vi "Stepper System Control.vi"() -> ()   [LabVIEW 2018]
uses:
  <vilib>/LabVIEW Interface for Arduino/LabVIEW Interface for Arduino.lvlib
panel:
  in  "zero bottom":bool
  in  "stop program":bool
  in  "return to start":bool
  out "Current position":dbl
  in  "move":bool
  in  "Distance to go (mm)":dbl
  in  "Set speed (steps/s)":dbl min=0.0 max=140.0
  in  "turn":bool
  in  "Serial Port":refnum<visa-resource-name>
  in  "zero top":bool
  # "Returns to lowest position."
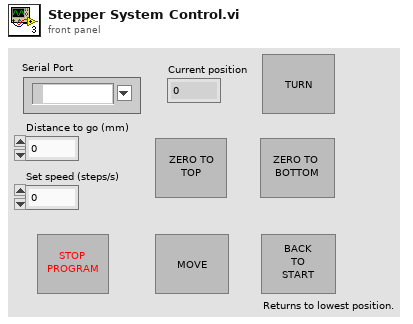
[diagram p1: front panel]
types:
  T1 = typedef "LabVIEW Interface for Arduino.lvlib/Arduino Resource.ctl" = cluster{"VISA resource":refnum<visa-resource-name>, "Board Type":T2, "Connection Type":enum8{"USB / Serial"}, "Bytes Per Packet (15)":u8}
  T2 = typedef "LabVIEW Interface for Arduino.lvlib/Board Type.ctl" = enum16{"Uno", "Dimuelanove w/Atmega 328", "Mega 2560"}
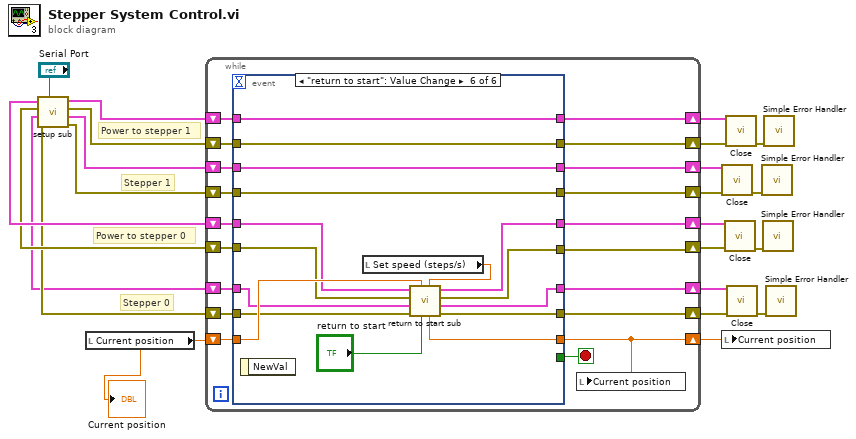
[diagram p0: block diagram]
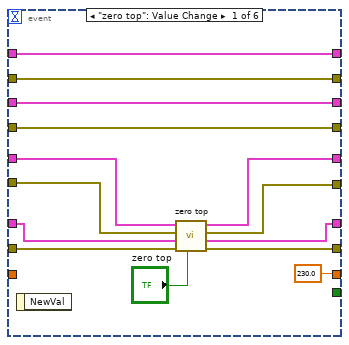
[diagram p2: hidden frame]
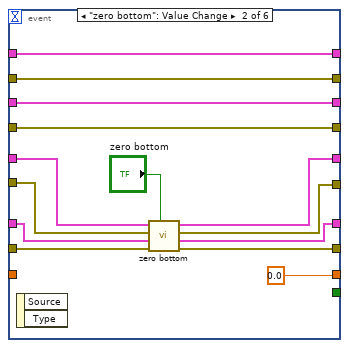
[diagram p3: hidden frame]
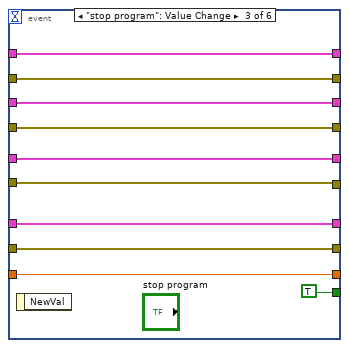
[diagram p4: hidden frame]
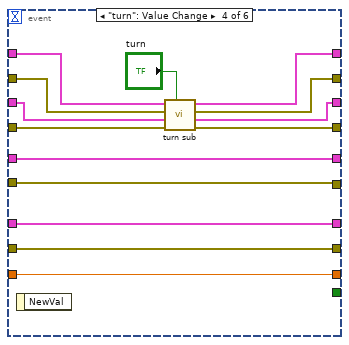
[diagram p5: hidden frame]
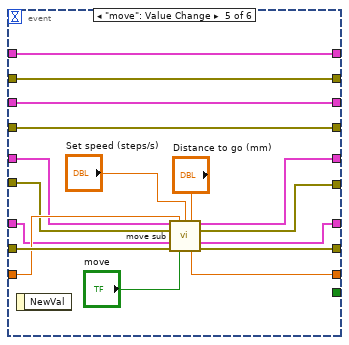
[diagram p6: hidden frame]
diagram:
  # "Power to stepper 0"
  # "Power to stepper 1"
  # "Stepper 1"
  # "Stepper 0"
  n1 = call "setup sub.vi"("Serial port in"="Serial Port") -> ("Stepper 1 error out"=w9:errorcluster, "Stepper 1 out"=w8:T1, "Pin 8 error out"=w1:errorcluster, "Pin 8 out"=w2:T1, "Stepper 0 error out"=w4:errorcluster, "Stepper 0 out"=w3:T1, "Pin 2 error out"=w6:errorcluster, "Pin 2 out"=w7:T1)  [unwired: 3 in]
  n2 = local read "Current position"() -> (w13:dbl)
  "Current position" <- w13
  n3 = while {
    shift-right: [w32] -> w16
    shift-left: w3 -> [w42]
    shift-right: [w33] -> w17
    shift-left: w4 -> [w41]
    shift-right: [w31] -> w15
    shift-left: w8 -> [w40]
    shift-right: [w34] -> w18
    shift-left: w9 -> [w39]
    shift-right: [w36] -> w20
    shift-left: w7 -> [w38]
    shift-right: [w35] -> w19
    shift-left: w6 -> [w37]
    shift-right: [w28] -> w14
    shift-left: w13 -> [w30]
    shift-right: [w27] -> w11
    shift-left: w2 -> [w24]
    shift-right: [w26] -> w10
    shift-left: w1 -> [w25]
    stop <- w29 stop-if-true
    n4 = event shown="[5] \"return to start\": Value Change" {
      selector: _ -> [_ _ _ _ _ _]
      dyn-events: _ -> [_ _ _ _ _ _]
      timeout: _ -> [_ _ _ _ _ _]
      tunnel: w42 -> [w53 w68 w74 w88 w101 w124]
      tunnel: w41 -> [w55 w69 w73 w87 w110 w123]
      tunnel: w40 -> [w51 w59 w77 w91 w108 w120]
      tunnel: w39 -> [w50 w60 w76 w94 w107 w119]
      tunnel: w38 -> [w48 w65 w79 w86 w104 w115]
      tunnel: w37 -> [w49 w66 w78 w85 w105 w116]
      tunnel: [w46 w64 w79 w86 w106 w117] -> w36
      tunnel: [w47 w63 w78 w85 w98 w118] -> w35
      tunnel: [w50 w60 w76 w92 w107 w119] -> w34
      tunnel: [w54 w70 w73 w87 w99 w121] -> w33
      tunnel: [w52 w67 w74 w88 w100 w122] -> w32
      tunnel: [w51 w59 w77 w90 w108 w120] -> w31
      tunnel: w30 -> [_ _ w75 w89 w109 w125]
      tunnel: [230.0 0.0 w75 w89 w97 w126] -> w28
      tunnel: [_ _ TRUE _ _ _] -> w29
      tunnel: [w44 w57 w71 w84 w95 w112] -> w27
      tunnel: [w45 w58 w72 w83 w96 w113] -> w26
      tunnel: w25 -> [w45 w58 w72 w82 w96 w113]
      tunnel: w24 -> [w44 w57 w71 w81 w95 w112]
      event "zero top": Value Change {
        n5 = event-data() -> ()  [unwired: 1 in, 1 out]
        n6 = call "zero top.vi"("zero"="zero top", "Stepper 0 error in"=w55, "Stepper 0 in"=w53, "Pin 2 error in"=w49, "Pin 2 in"=w48) -> ("Stepper 0 error out"=w54:errorcluster, "Stepper 0 out"=w52:T1, "Pin 2 error out"=w47:errorcluster, "Pin 2 out"=w46:T1)  [unwired: 3 in]
      }
      event "zero bottom": Value Change {
        n7 = event-data() -> ()  [unwired: 1 in, 2 out]
        n8 = call "zero bottom.vi"("zero"="zero bottom", "Stepper 0 error in"=w69, "Stepper 0 in"=w68, "Pin 2 error in"=w66, "Pin 2 in"=w65) -> ("Stepper 0 error out"=w70:errorcluster, "Stepper 0 out"=w67:T1, "Pin 2 error out"=w63:errorcluster, "Pin 2 out"=w64:T1)  [unwired: 3 in]
      }
      event "stop program": Value Change {
        n9 = event-data() -> ()  [unwired: 1 in, 1 out]
      }
      event "turn": Value Change {
        n10 = event-data() -> ()  [unwired: 1 in, 1 out]
        n11 = call "turn sub.vi"("turn Button"="turn", "Stepper 1 error in"=w94, "Stepper 1 in"=w91, "Pin 12 error in"=w82, "Pin 12 in"=w81) -> ("Stepper 1 error out"=w92:errorcluster, "Stepper 1 out"=w90:T1, "Pin 12 error out"=w83:errorcluster, "Pin 12 out"=w84:T1)  [unwired: 3 in]
      }
      event "move": Value Change {
        n12 = event-data() -> ()  [unwired: 1 in, 1 out]
        n13 = call "move sub.vi"("Pin 2 in"=w104, "Current position in"=w109, "Set speed"="Set speed (steps/s)", "mm to go"="Distance to go (mm)", "Pin 2 error in"=w105, "Stepper 0 in"=w101, "Stepper 0 error in"=w110, "Move"="move") -> ("Pin 2 out"=w106:T1, "Pin 2 error out"=w98:errorcluster, "Stepper 0 out"=w100:T1, "Current position out"=w97:dbl, "Stepper 0 error out"=w99:errorcluster)  [unwired: 3 in]
      }
      event "return to start": Value Change {
        n14 = event-data() -> ()  [unwired: 1 in, 1 out]
        n15 = local read "Set speed (steps/s)"() -> (w114:dbl)
        n16 = call "return to start sub.vi"("Set speed"=w114, "Return to start"="return to start", "Current position in"=w125, "Stepper 0 error in"=w123, "Stepper 0 in"=w124, "Pin 2 error in"=w116, "Pin 2 in"=w115) -> ("Stepper 0 error out"=w121:errorcluster, "Stepper 0 out"=w122:T1, "Pin 2 error out"=w118:errorcluster, "Pin 2 out"=w117:T1, "Current position out"=w126:dbl)
      }
    }
    n17 = local write "Current position"(w28) -> ()
  }
  n18 = call <vilib>:"Close.vi"("Arduino Resource"=w15, "error in"=w18) -> ("error out"=w22:errorcluster)  [unwired: 13 in]
  n19 = local write "Current position"(w14) -> ()
  n20 = call <vilib>:"Close.vi"("Arduino Resource"=w20, "error in"=w19) -> ("error out"=w21:errorcluster)  [unwired: 13 in]
  n21 = call <vilib>:"Close.vi"("Arduino Resource"=w11, "error in"=w10) -> ("error out"=w12:errorcluster)  [unwired: 13 in]
  n22 = call <vilib>:"Close.vi"("Arduino Resource"=w16, "error in"=w17) -> ("error out"=w23:errorcluster)  [unwired: 13 in]
  n23 = call <vilib>:"Simple Error Handler.vi"("error in (no error)"=w22) -> ()  [unwired: 4 in, 5 out]
  n24 = call <vilib>:"Simple Error Handler.vi"("error in (no error)"=w21) -> ()  [unwired: 4 in, 5 out]
  n25 = call <vilib>:"Simple Error Handler.vi"("error in (no error)"=w12) -> ()  [unwired: 4 in, 5 out]
  n26 = call <vilib>:"Simple Error Handler.vi"("error in (no error)"=w23) -> ()  [unwired: 4 in, 5 out]
